vi "svl_Equivalent Continuous Level (N Ch).vi"(8 "error in (no error)":errorcluster, 9 "processing state":T1(ring), 11 "scaled signals [EU]":waveform(dbl)[](array[waveform])) -> (0 "error out":errorcluster, 3 "equivalent continuous levels [EU^2 rms]":dbl[](array[numeric]) format="%.2f")   [LabVIEW 2017]
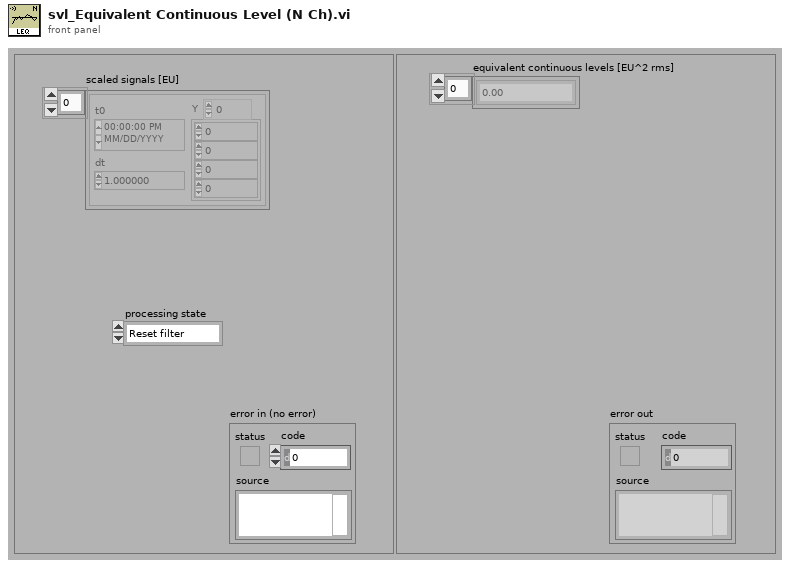
[diagram p1: front panel]
types:
  T1 = enum16{"Reset filter", "Restart averaging", "Continue processing"}
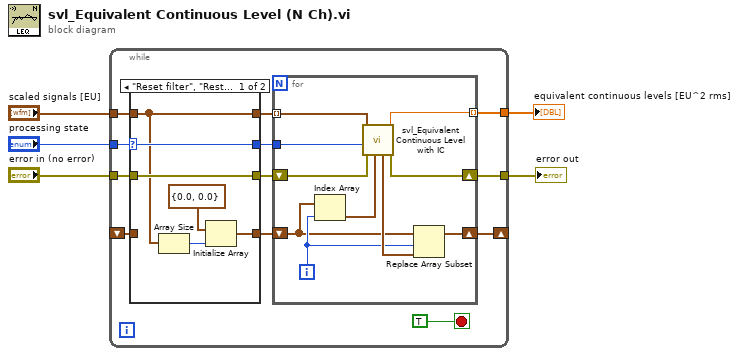
[diagram p0: block diagram]
diagram:
  n1 = while {
    tunnel: [w10] -> w1
    tunnel: [w11] -> w2
    shift-left: _ -> [w13]
    shift-right: [w16] -> _
    tunnel: "error in (no error)" -> [w7]
    tunnel: "scaled signals [EU]" -> [w9]
    tunnel: "processing state" -> [w15]
    stop <- TRUE stop-if-true
    n2 = case shown="\"Reset filter\", \"Restart averaging\", Default" w15 {
      selector: w15 -> [w23 w27]
      tunnel: [w23 w27] -> w14
      tunnel: w13 -> [_ w26]
      tunnel: [w21 w26] -> w12
      tunnel: w9 -> [w19 w25]
      tunnel: [w19 w25] -> w8
      tunnel: [w20 w24] -> w6
      tunnel: w7 -> [w20 w24]
      frame "Reset filter", "Restart averaging", Default {
        n3 = Array Size(array=w19) -> (size(s)=w18:i32)
        n4 = Initialize Array(cluster{"squaredSum":dbl, "squaredSum 2":dbl} {"squaredSum"=0.0, "squaredSum 2"=0.0} ("Final state"), w18) -> (w21:cluster{"squaredSum":dbl, "squaredSum 2":dbl}[])
      }
      frame "Continue processing" {
      }
    }
    n5 = for {
      tunnel: w8 -> [w28] mode=indexing
      shift-right: [w37] -> w16
      shift-left: w12 -> [w34]
      shift-right: [w31] -> w10
      shift-left: w6 -> [w32]
      tunnel: w14 -> [w29]
      tunnel: [w30] -> w11 mode=indexing
      i -> [w35]
      n6 = Index Array(array=w34, index=w35) -> (element=w33:cluster{"squaredSum":dbl, "squaredSum 2":dbl})
      n7 = call <vilib>:"svl_Equivalent Continuous Level with IC.vi"("state in"=w33, "error in (no error)"=w32, "processing state"=w29, "scaledSignal"=w28) -> ("error out"=w31:errorcluster, "Numeric"=w30:dbl, "state out"=w36:cluster{dbl, dbl})  [unwired: 5 in]
      n8 = Replace Array Subset(array=w34, new element=w36, index=w35) -> (w37:cluster{"squaredSum":dbl, "squaredSum 2":dbl}[])
    }
  }
  "equivalent continuous levels [EU^2 rms]" <- w2
  "error out" <- w1
